vi "mToPixels-MissionControl.vi"(2 "Arena Pixel Dim":i32[](array[numeric])=[1000, 512], 3 "y (m)":dbl, 4 "x (m)":dbl) -> (0 "y (pixels)":dbl, 1 "x (pixels)":dbl)   [LabVIEW 2015, in "MissionControl2017.lvlib" / "SubVIs - MissionControl2017.lvlib"]
uses:
  SubVIs - MissionControl2017.lvlib
  Navigation2017.lvlib
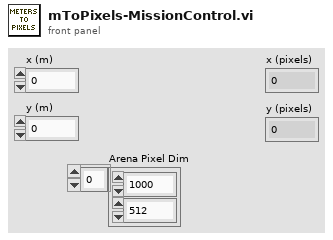
[diagram p1: front panel]
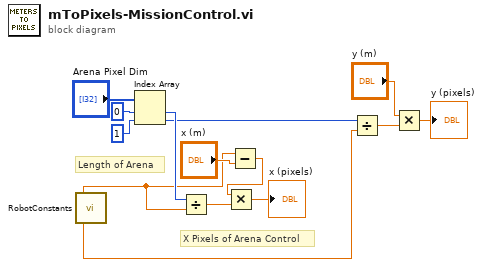
[diagram p0: block diagram]
diagram:
  # "X Pixels of Arena Control"
  # "Length of Arena"
  n1 = call "RobotConstants.vi"() -> ("Arena Width (m)"=w2:dbl, "Arena Height (m)"=w10:dbl)  [unwired: 3 out]
  n2 = Index Array(array="Arena Pixel Dim", index #1=0 ("index"), index #2=1) -> (element #1=w11:i32, element #2=w8:i32)
  n3 = Divide(x=w11, y=w2) -> (x/y=w13:dbl)
  n4 = Subtract(x=w2, y="x (m)") -> (x-y=w1:dbl)
  n5 = Multiply(x=w1, y=w13) -> (x*y=→"x (pixels)":dbl)
  n6 = Divide(x=w8, y=w10) -> (x/y=w6:dbl)
  n7 = Multiply(x="y (m)", y=w6) -> (x*y=→"y (pixels)":dbl)
